vi "Build Events.vi"(8 "error in (no error)":errorcluster, 11 "CI Project in":refnum<class "CI Project.lvclass">) -> (0 "error out":errorcluster, 2 "Build Events":refnum<user-event>, 3 "CI Project out":refnum<class "CI Project.lvclass">)   [LabVIEW 2014, in "CI Project.lvclass"]
uses:
  CI Project.lvclass
  CI Project.lvclass/CI Project.ctl
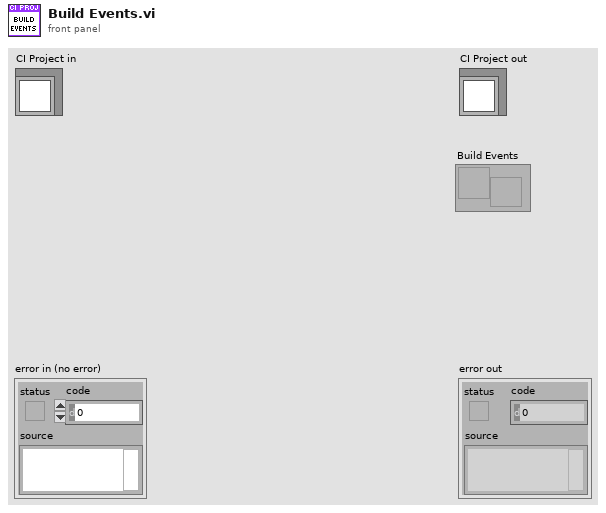
[diagram p1: front panel]
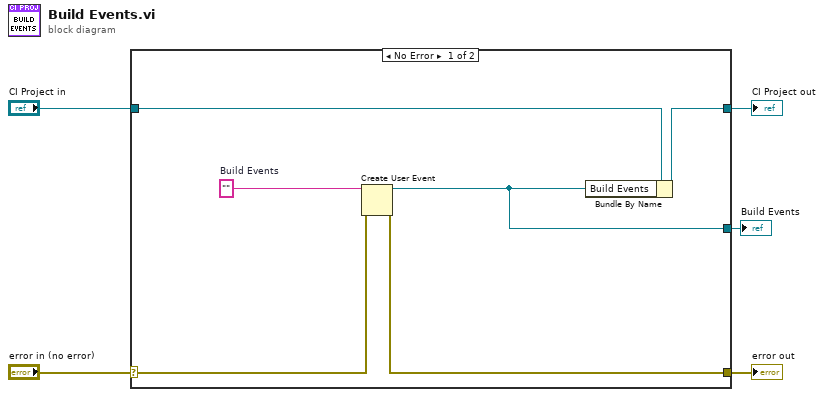
[diagram p0: block diagram]
diagram:
  n1 = case shown="No Error" "error in (no error)" {
    selector: "error in (no error)" -> [w8 w13]
    tunnel: [w7 w13] -> w4
    tunnel: [w9 w12] -> w2
    tunnel: "CI Project in" -> [w10 w12]
    tunnel: [w6 _] -> w1
    frame No Error {
      w11 = ""  # Build Events
      n2 = Create User Event(user event datatype=w11, error in=w8) -> (user event=w6:refnum<user-event>, error out=w7:errorcluster)
      n3 = Bundle By Name(cluster=w10, "Build Events"=w6) -> (w9:refnum<class "CI Project.lvclass">)
    }
    frame Error {
    }
  }
  "error out" <- w4
  "CI Project out" <- w2
  "Build Events" <- w1
